vi "Generarea_unui_nr_aleator.vi"() -> ()   [LabVIEW 2019]
panel:
  out "Afisare numar aleator":dbl(graph)
  in  "Intrare limita H":dbl(slide) scale=0.0..10.0
  # "Generarea unui numãr aleator între 0 si H"
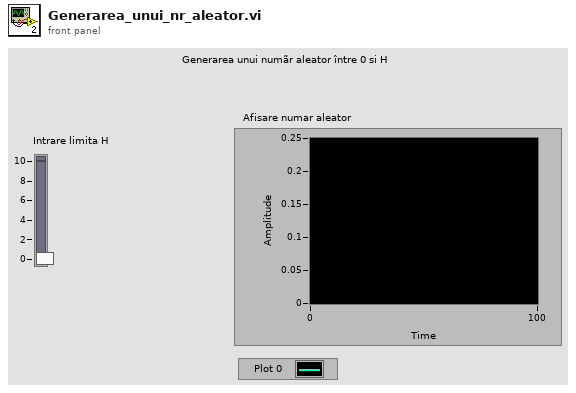
[diagram p1: front panel]
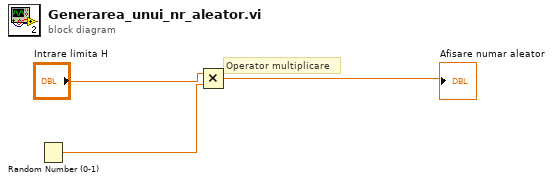
[diagram p0: block diagram]
diagram:
  # "Operator multiplicare"
  n1 = Random Number (0-1)() -> (number: 0 to 1=w2:dbl)
  n2 = Multiply(x="Intrare limita H", y=w2) -> (x*y=→"Afisare numar aleator":dbl)
